vi "int_P_F.vi"(9 "INT":i32, 10 "32INT in":i32[](array[numeric])) -> (2 "pass":bool)   [LabVIEW 2020]
uses:
  933eea8f-aa5f-4b01-874f-acf024cac0e1.vi
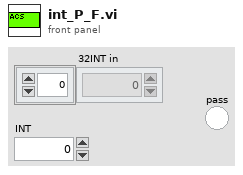
[diagram p1: front panel]
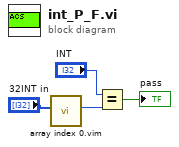
[diagram p0: block diagram]
diagram:
  n1 = call "array index 0.vim"("32INT in"="32INT in") -> ("Numeric"=w2:i32)  [unwired: 10 in]
  n2 = Equal?(x="INT", y=w2) -> (x = y?=→"pass":bool)
